vi "Example context menu.vi"   [LabVIEW 2013]
uses:
  PopUp Menu/TD_PopUp Menu_Items.ctl
  PopUp Menu/TD_PopUp Menu_Flags.ctl
panel:
  # "Press play and then right click anywhere on the window..."
types:
  T1 = typedef "TD_PopUp Menu_Items.ctl" = cluster{"ItemName":string, "Item Tag":string, "Parent":string, "uFlags":T2[]}
  T2 = typedef "TD_PopUp Menu_Flags.ctl" = u32
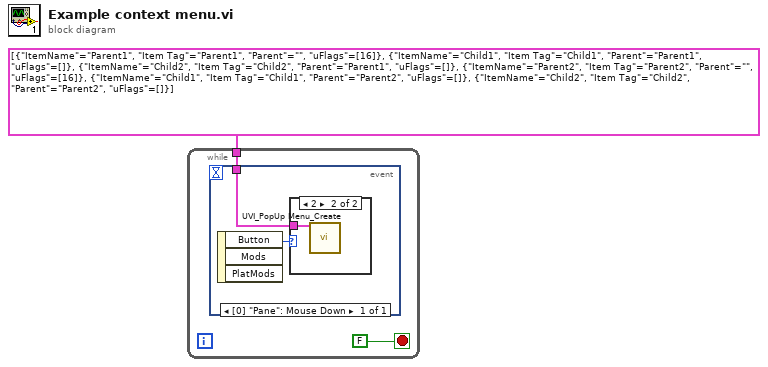
[diagram p0: block diagram]
diagram:
  n1 = while {
    tunnel: T1[] [{"ItemName"="Parent1", "Item Tag"="Parent1", "Parent"="", "uFlags"=[16]}, {"ItemName"="Child1", "Item Tag"="Child1", "Parent"="Parent1", "uFlags"=[]}, {"ItemName"="Child2", "Item Tag"="Child2", "Parent"="Parent1", "uFlags"=[]}, {"ItemName"="Parent2", "Item Tag"="Parent2", "Parent"="", "uFlags"=[16]}, {"ItemName"="Child1", "Item Tag"="Child1", "Parent"="Parent2", "uFlags"=[]}, {"ItemName"="Child2", "Item Tag"="Child2", "Parent"="Parent2", "uFlags"=[]}] ("PopUpMenuItems") -> [w3]
    stop <- FALSE stop-if-true
    n2 = event shown="[0] \"Pane\": Mouse Down" {
      selector: _ -> [_]
      dyn-events: _ -> [_]
      timeout: _ -> [_]
      tunnel: w3 -> [w4]
      event Mouse Down {
        n3 = event-data() -> ("Button"=w5:u16)  [unwired: 3 out]
        n4 = case shown="2" w5 {
          tunnel: w4 -> [_ w6]
          frame 0, Default {
          }
          frame 2 {
            n5 = call "UVI_PopUp Menu_Create.vi"("PopUpMenuItems"=w6) -> ()  [unwired: 4 in, 11 out]
          }
        }
      }
    }
  }
